vi "Configure Digital IO Line Mode.vi"(6 "Digital IO Mode (0: In)":T1(ring), 8 "error in (no error)":errorcluster, 9 "Digital IO Trigger Type (0: Digital)":enum16{"Digital", "Trigger", "Synchronous"}(ring), 10 "Digital IO Line (1)":u32 min=1 max=6 step=1, 11 "VISA resource name":refnum<visa-resource-name>) -> (0 "error out":errorcluster, 3 "VISA resource name out":refnum<visa-resource-name>)   [LabVIEW 2009, in "Keithley DMM7510.lvlib"]
doc: "This VI sets the mode of the digital I/O line to be a digital line, trigger line, or synchronous line and sets the line to be input, output, or open-drain."
uses:
  Keithley DMM7510.lvlib
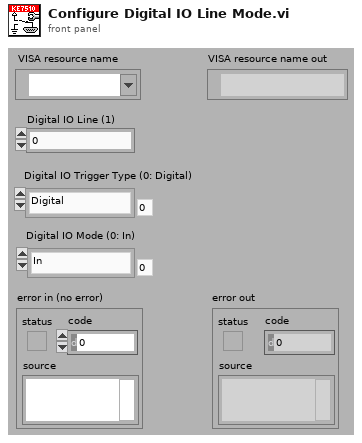
[diagram p1: front panel]
types:
  T1 = enum16{"In", "Out", "Open Drain", "Acceptor", "Master"}
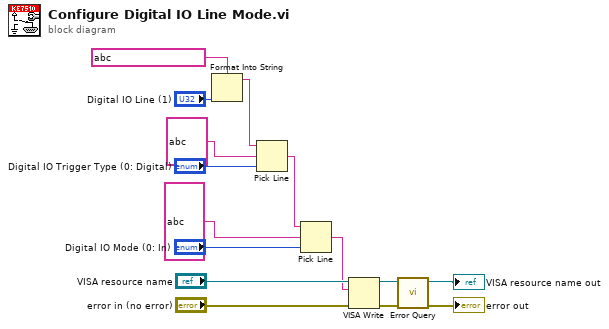
[diagram p0: block diagram]
diagram:
  n1 = Format Into String(format string=string ?, "Digital IO Line (1)") -> (resulting string=w6:string)  [unwired: 2 in, 1 out]
  n2 = Pick Line(string ("")=w6, multi-line string=string ?, line index="Digital IO Trigger Type (0: Digital)") -> (output string=w2:string)
  n3 = Pick Line(string ("")=w2, multi-line string=string ?, line index="Digital IO Mode (0: In)") -> (output string=w1:string)
  n4 = VISA Write(VISA resource name="VISA resource name", write buffer=w1, error in (no error)="error in (no error)") -> (VISA resource name out=w13:refnum<visa-resource-name>, error out=w10:errorcluster)  [unwired: 1 out]
  n5 = call "Error Query.vi"("error in (no error)"=w10, "VISA resource name"=w13) -> ("error out"=→"error out":errorcluster, "VISA resource name out"=→"VISA resource name out":refnum<visa-resource-name>)  [unwired: 6 in, 2 out]
